vi "macro_Elevator_Sim_Execute.vi"() -> ()   [LabVIEW 2019, in "Trajectory_Library.lvlib"]
uses:
  Trajectory_Library.lvlib
  Enum/DCMOTOR_TYPES_ENUM.ctl
  BatterySim_CalculateLoadedBatteryVoltage.vi
panel:
  in  "Motor Dmd (CO)":dbl
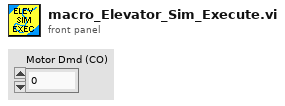
[diagram p1: front panel]
types:
  T1 = typedef "Trajectory_Library.lvlib/DCMOTOR_TYPES_ENUM.ctl" = enum16{"CIM", "AndyMark 9015", "Andy Mark RS 775 125", "Bag", "BaneBots RS 550", "BaneBots RS 775", "Falcon 500", "Mini CIM", "NEO", "NEO 550", "Romi BuiltIn", "Vex 775 Pro", "Snow Blower AM 2235A", "Bosch Seat AM 3493"}
  T2 = typedef "Trajectory_Library.lvlib/LINEAR_SYSTEM_ID_ELEVATOR_MODEL.CTL" = cluster{"DCMOTOR_TYPES":T1, "Num Motors":i32, "WinchRadias_Meters":dbl, "mass_Kg":dbl, "Gearing":dbl}
  T3 = typedef "Trajectory_Library.lvlib/ELEVATOR_SIM_SIMULATION_PARAMS.ctl" = cluster{"MinHeight_Meters":dbl, "MaxHeight_Meters":dbl, "Measurment StdDev":dbl, "SimulateGravity":bool}
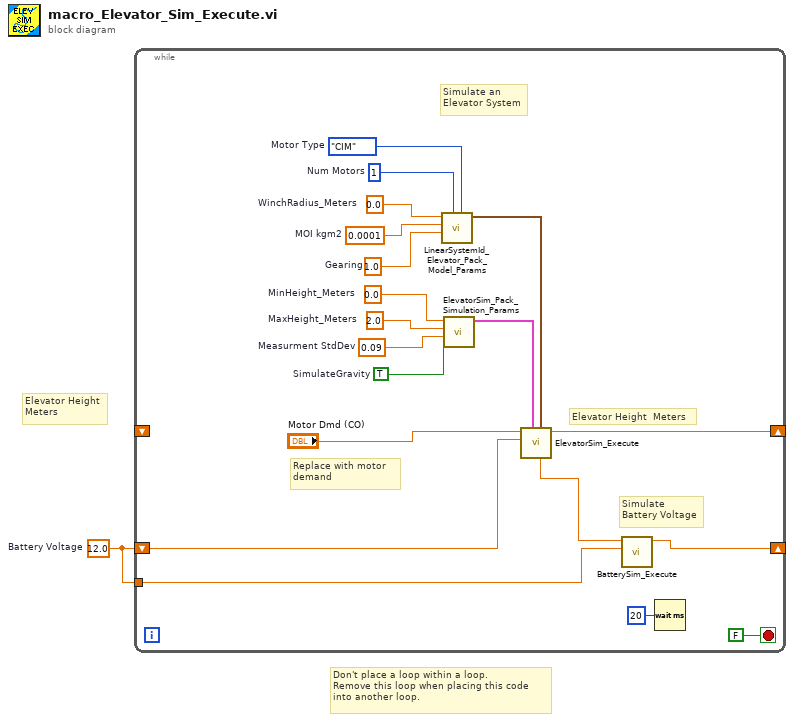
[diagram p0: block diagram]
diagram:
  w1 = 12.0  # Battery Voltage
  # "Don't place a loop within a loop. \nRemove this loop when placing this code\ninto another loop."
  # "Elevator Height\nMeters"
  n1 = while {
    shift-right: [w14] -> _
    shift-left: w1 -> [w4]
    shift-right: [w13] -> _
    shift-left: _ -> [_]
    tunnel: w1 -> [w2]
    stop <- FALSE stop-if-true
    w8 = 0.0  # MinHeight_Meters
    w9 = 2.0  # MaxHeight_Meters
    w10 = 0.09  # Measurment StdDev
    w11 = TRUE  # SimulateGravity
    w12 = 0.0  # WinchRadius_Meters
    w17 = 1.0  # Gearing
    w18 = 0.0001  # MOI kgm2
    w19 = 1  # Num Motors
    w20 = DCMOTOR_TYPES_ENUM."CIM"  # Motor Type
    # "Elevator Height  Meters"
    # "Replace with motor \ndemand"
    # "Simulate\nBattery Voltage"
    # "Simulate an \nElevator System"
    n2 = call "LinearSystemId_Elevator_Pack_Model_Params.vi"("DCMOTOR_TYPES"=w20, "Num Motors"=w19, "Gearing"=w17, "mass_Kg"=w18, "WinchRadius_Meters"=w12) -> ("Elevator_Model _Params"=w7:T2)  [unwired: 6 in]
    n3 = call "ElevatorSim_Pack_Simulation_Params.vi"("SimulateGravity"=w11, "Measurment StdDev"=w10, "MaxHeight_Meters"=w9, "MinHeight_Meters"=w8) -> ("ElevatorSim_Simulation _Params"=w6:T3)  [unwired: 7 in]
    n4 = call "ElevatorSim_Execute.vi"("LinearSystemID_Elevator_Model _Params"=w7, "ElevatorSim_Simulation _Params"=w6, "Battery Volts"=w4, "Motor Dmd"="Motor Dmd (CO)") -> ("ElevatorHeight_Meters"=w13:dbl, "Motor Current"=w3:dbl)  [unwired: 2 in, 4 out]
    n5 = call "BatterySim_Execute.vi"("Nominal Battery Voltage"=w2, "Current"=w3) -> ("Voltage"=w14:dbl)  [unwired: 9 in]
    n6 = Wait (ms)(milliseconds to wait=u32 20) -> ()  [unwired: 1 out]
  }
